vi "Calc_ideal_fid_locations_from_angles.vi"(9 "r":dbl, 11 "Array in":dbl[](array[numeric])) -> (3 "Array out":T1[](array[typedef]))   [LabVIEW 2011]
uses:
  cm2nm_coordinate_information_v2.ctl
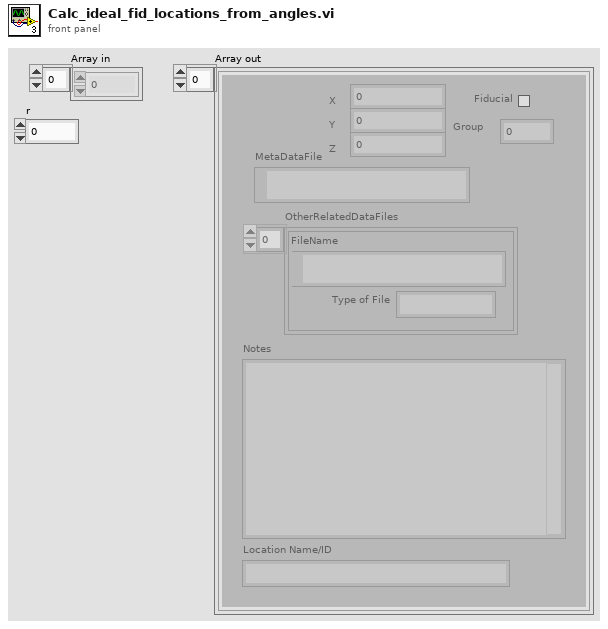
[diagram p1: front panel]
types:
  T1 = typedef "cm2nm_coordinate_information_v2.ctl" = cluster{"MetaDataFile":path, "X":dbl, "Y":dbl, "Z":dbl, "Group":i32, "Rotation":dbl[unit], "Fiducial":bool, "Magnification":dbl, "Working_Distance":dbl, "Notes":string, "Location Name/ID":string, "OtherRelatedDataFiles":cluster{"Type of File":string, "FileName":path}[], "Available":bool}
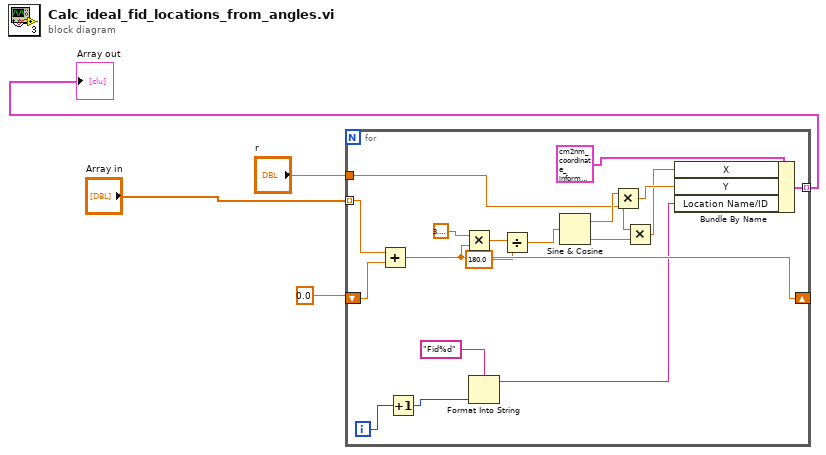
[diagram p0: block diagram]
diagram:
  n1 = for {
    tunnel: "Array in" -> [w22] mode=indexing
    shift-right: [w20] -> _
    shift-left: 0.0 -> [w21]
    tunnel: [w6] -> w4 mode=indexing
    tunnel: "r" -> [w5]
    i -> [w12]
    n2 = Add(x=w22, y=w21) -> (x+y=w20:dbl)
    n3 = Increment(x=w12) -> (x+1=w11:i32)
    n4 = Multiply(x=3.141592653589793, y=w20) -> (x*y=w18:dbl)
    n5 = Format Into String(format string="Fid%d", w11) -> (resulting string=w7:string)  [unwired: 2 in, 1 out]
    n6 = Divide(x=w18, y=180.0) -> (x/y=w16:dbl)
    n7 = Sine & Cosine(0:w16) -> (1:w15:dbl, 2:w14:dbl)
    n8 = Multiply(x=w15, y=w5) -> (x*y=w9:dbl)
    n9 = Multiply(x=w5, y=w14) -> (x*y=w8:dbl)
    n10 = Bundle By Name(cluster=T1 {"MetaDataFile"=path "", "X"=8.636, "Y"=0.0, "Z"=0.0, "Group"=10, "Rotation"=0.0, "Fiducial"=TRUE, "Magnification"=0.0, "Working_Distance"=0.0, "Notes"="", "Location Name/ID"="Fid1", "OtherRelatedDataFiles"=[], "Available"=FALSE} ("Cluster"), "X"=w8, "Y"=w9, "Location Name/ID"=w7) -> (w6:T1)
  }
  "Array out" <- w4
